vi "Fin_init.vi"(8 "Error In":errorcluster, 11 "Fin Arrangement (SORTED)":u8[](array[numeric])) -> (0 "Error Out":errorcluster)   [LabVIEW 2013]
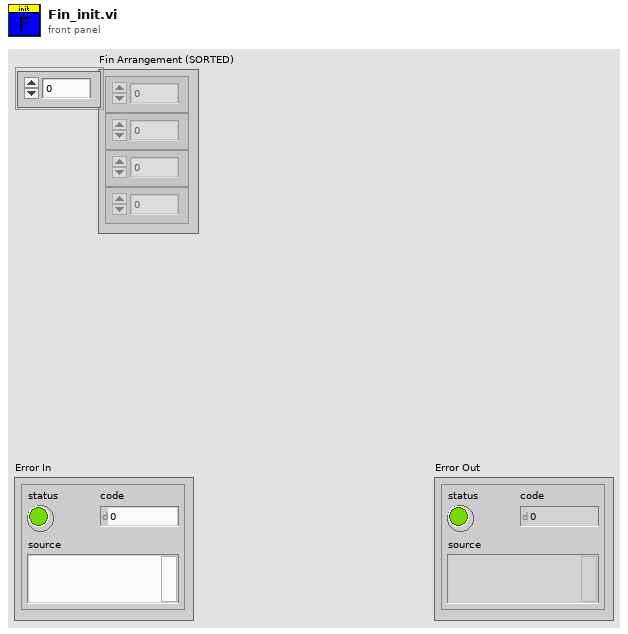
[diagram p1: front panel]
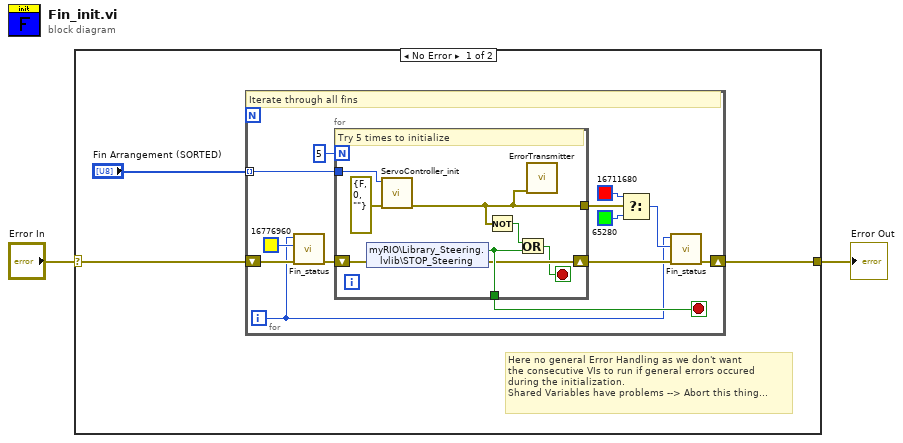
[diagram p0: block diagram]
diagram:
  n1 = case shown="No Error" "Error In" {
    selector: "Error In" -> [w4 w27]
    tunnel: [w3 w27] -> w1
    frame No Error {
      # "Here no general Error Handling as we don't want\nthe consecutive VIs to run if general errors occured\nduring the initialization.\nShared Variables have problems --> Abort this thing..."
      n2 = for {
        tunnel: "Fin Arrangement (SORTED)" -> [w16] mode=indexing
        shift-right: [w7] -> w3
        shift-left: w4 -> [w9]
        i -> [w6]
        stop <- w11 stop-if-true
        # "Iterate through all fins"
        n3 = call "Fin_status.vi"("Error In"=w9, "Round Color Box"=u32 16776960, "Fin Index"=w6) -> ("Error Out"=w10:errorcluster)  [unwired: 8 in]
        n4 = for {
          N: 5 -> [_]
          tunnel: w16 -> [w26]
          tunnel: [w21] -> w12
          tunnel: [w25] -> w11
          shift-right: [w20] -> w8
          shift-left: w10 -> [w22]
          stop <- w19 stop-if-true
          # "Try 5 times to initialize"
          n5 = shared-variable "myRIO\\Library_Steering.lvlib\\STOP_Steering"(error in=w22) -> (w25:bool, error out=w20:errorcluster)
          n6 = call "ServoController_init.vi"("Error In"=errorcluster {"status"=FALSE, "code"=0, "source"=""}, "Servo Controller Index"=w26) -> ("Error Out"=w21:errorcluster)  [unwired: 9 in]
          n7 = Not(x=w21) -> (.not. x?=w24:bool)
          n8 = Or(x=w24, y=w25) -> (x .or. y?=w19:bool)
          n9 = call "ErrorTransmitter.vi"("Error In"=w21) -> ()  [unwired: 10 in, 1 out]
        }
        n10 = Select(t=u32 16711680 ("Round Color Box"), s=w12, f=u32 65280 ("Round Color Box")) -> (s? t:f=w13:u32)
        n11 = call "Fin_status.vi"("Error In"=w8, "Round Color Box"=w13, "Fin Index"=w6) -> ("Error Out"=w7:errorcluster)  [unwired: 8 in]
      }
    }
    frame Error {
    }
  }
  "Error Out" <- w1
